vi "Simple Video.vi"() -> ()   [LabVIEW 2014]
doc: "Very simple example showing how to use the base VIs to control the AR Drone and receive and display video data."
uses:
  Resources/Global.vi
panel:
  out "x-y":u32
  in  "milliseconds to wait":u32=25
  out "error out 3":errorcluster
  out "Video Stream 2":picture
  # "Do NOT un this VI. Instead run \"AR.Drone MAIN.vi\" and select the name of this VI in the dop-down menu at the Steup tab"
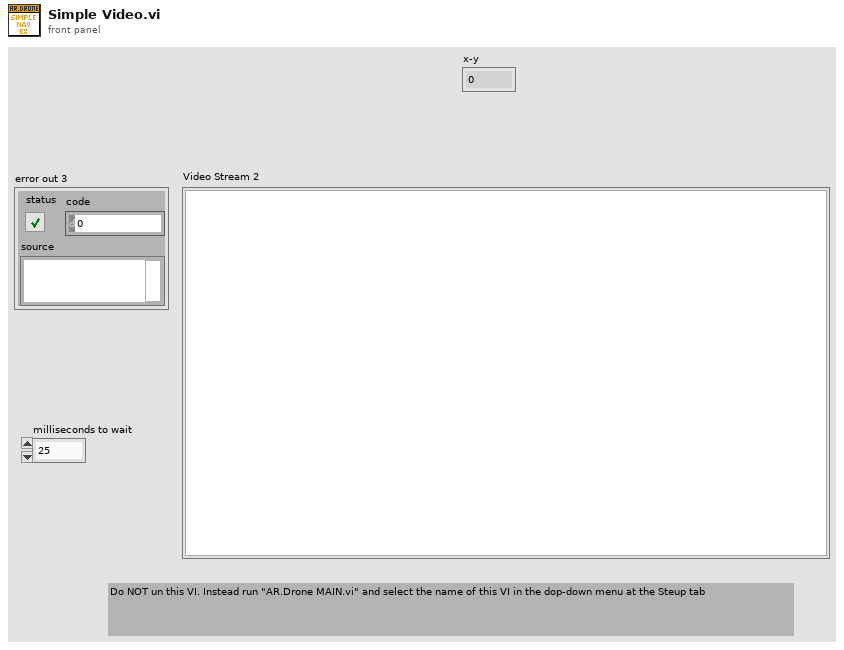
[diagram p1: front panel]
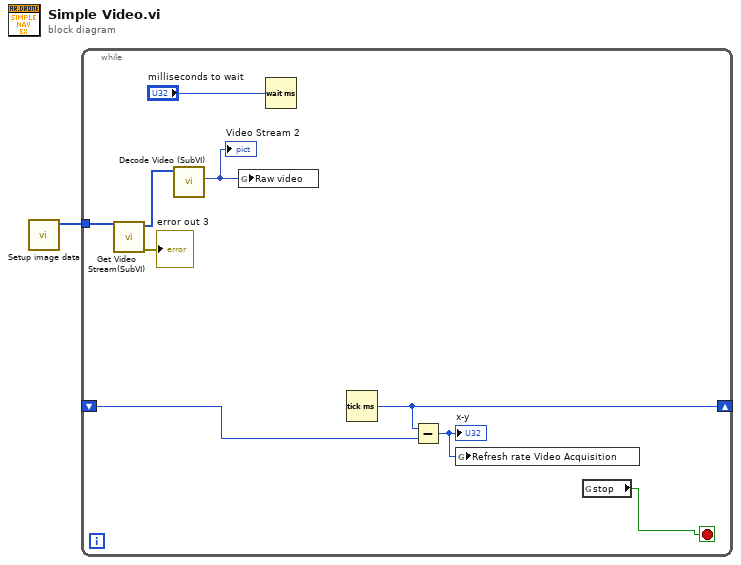
[diagram p0: block diagram]
diagram:
  n1 = call "Setup image data.vi"() -> ("Array"=w1:u8[])  [unwired: 11 in]
  n2 = while {
    tunnel: w1 -> [w5]
    shift-right: [w4] -> _
    shift-left: _ -> [w3]
    stop <- w6 stop-if-true
    n3 = call "Get Video Stream(SubVI).vi"("ImgData 2"=w5) -> ("error out"=→"error out 3":errorcluster, "ImgData"=w9:u8[])  [unwired: 9 in]
    n4 = call "Decode Video (SubVI).vi"("ImgData"=w9) -> ("new picture"=w8:picture)  [unwired: 9 in, 1 out]
    "Video Stream 2" <- w8
    n5 = global write "Global.vi" "Raw video"(w8) -> ()
    n6 = Wait (ms)(milliseconds to wait="milliseconds to wait") -> ()  [unwired: 1 out]
    n7 = Tick Count (ms)() -> (millisecond timer value=w4:u32)
    n8 = Subtract(x=w4, y=w3) -> (x-y=w2:u32)
    "x-y" <- w2
    n9 = global write "Global.vi" "Refresh rate Video Acquisition"(w2) -> ()
    n10 = global read "Global.vi" "stop"() -> (w6:bool)
  }
